vi "Read channel config.vi"(8 "error in (no error)":errorcluster, 11 "Runtime.Channel in":refnum<class "Runtime.Channel.lvclass">) -> (0 "error out":errorcluster, 2 "channel config":T1, 3 "Runtime.Channel out":refnum<class "Runtime.Channel.lvclass">)   [LabVIEW 2016, in "Data Sharing Framework.Runtime.lvlib" / "Runtime.Channel.lvclass"]
uses:
  Runtime.Channel.lvclass
  Typedefs/Channel Configuration.ctl
  <vilib>/NI Veristand/VeriStand Data/Typedefs/Typedefs.Data Types.ctl
  Runtime.Channel.lvclass/Runtime.Channel.ctl
  <vilib>/NI Veristand/VeriStand Data/VeriStand Data.lvlib
  Configuration.Channel/Configuration.Channel.lvclass
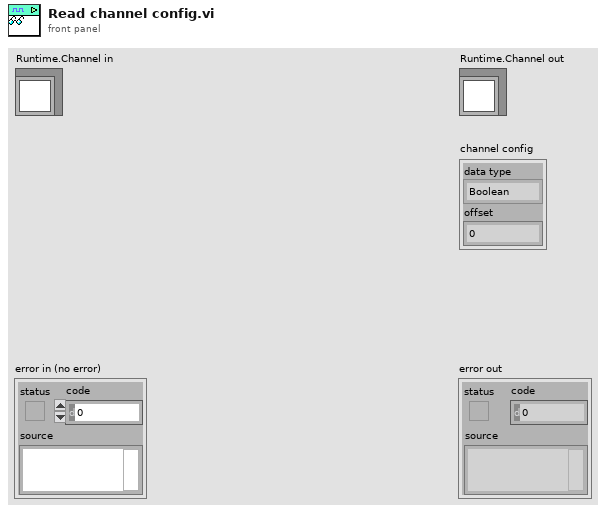
[diagram p1: front panel]
types:
  T1 = typedef "Data Sharing Framework.Configuration.lvlib/Configuration.Channel.lvclass/Channel Configuration.ctl" = cluster{"data type":T2, "offset":u64}
  T2 = typedef "VeriStand Data.lvlib/Typedefs.Data Types.ctl" = enum16{"Boolean", "Single", "Double", "I8", "I16", "I32", "I64", "U8", "U16", "U32", "U64"}
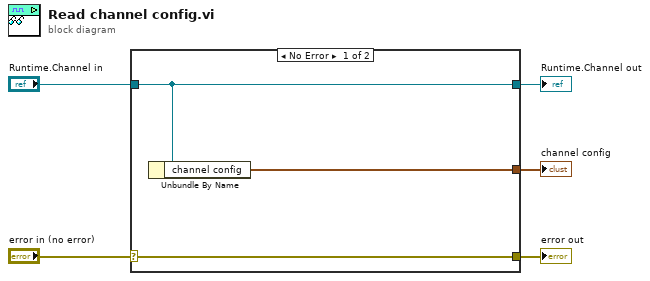
[diagram p0: block diagram]
diagram:
  n1 = case shown="No Error" "error in (no error)" {
    selector: "error in (no error)" -> [w8 w9]
    tunnel: [w8 w9] -> w4
    tunnel: [w7 w10] -> w2
    tunnel: "Runtime.Channel in" -> [w7 w10]
    tunnel: [w6 _] -> w1
    frame No Error {
      n2 = Unbundle By Name(w7) -> ("channel config"=w6:T1)
    }
    frame Error {
    }
  }
  "error out" <- w4
  "Runtime.Channel out" <- w2
  "channel config" <- w1
